vi "Output Build Result.vi"(8 "error in (no error)":errorcluster, 9 "Build Error":errorcluster, 10 "Built Path":path, 11 "CLI in":refnum<class "CLI.lvclass">) -> (0 "error out":errorcluster, 2 "Outputted String":string, 3 "CLI out":refnum<class "CLI.lvclass">)   [LabVIEW 2019]
uses:
  <vilib>/Wiresmith Technology/G CLI/CLI Class/CLI.lvclass
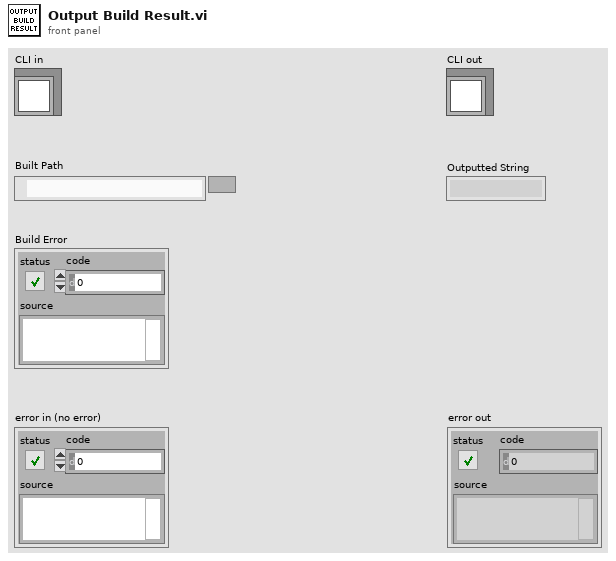
[diagram p1: front panel]
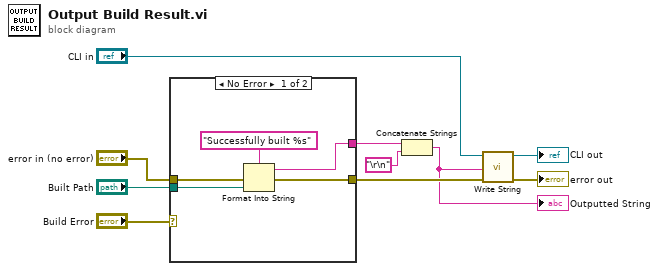
[diagram p0: block diagram]
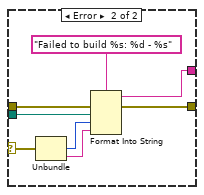
[diagram p2: hidden frame]
diagram:
  n1 = case shown="No Error" "Build Error" {
    selector: "Build Error" -> [_ w21]
    tunnel: "Built Path" -> [w15 w22]
    tunnel: [w13 w17] -> w3
    tunnel: [w12 w16] -> w6
    tunnel: "error in (no error)" -> [w11 w18]
    frame No Error {
      n2 = Format Into String(format string="Successfully built %s", error in=w11, w15) -> (resulting string=w13:string, error out=w12:errorcluster)  [unwired: 1 in]
    }
    frame Error {
      n3 = Unbundle(w21) -> ("code"=w20:i32, "source"=w19:string)  [unwired: 1 out]
      n4 = Format Into String(format string="Failed to build %s: %d - %s", error in=w18, w22, w20, w19) -> (resulting string=w17:string, error out=w16:errorcluster)  [unwired: 1 in]
    }
  }
  n5 = Concatenate Strings(w3, "\r\n") -> (w2:string)
  "Outputted String" <- w2
  n6 = call <vilib>:"Write String.vi"("error in (no error)"=w6, "Text to Write"=w2, "CLI in"="CLI in") -> ("error out"=→"error out":errorcluster, "CLI out"=→"CLI out":refnum<class "CLI.lvclass">)  [unwired: 7 in]
